vi "ET3500 - Read Program Parameters.vi"(4 "Sample/ch per Count":i32, 6 "Simulate":bool, 7 "ET3500 Status":refnum<vi>, 8 "error in (no error)":errorcluster, 9 "subVI (Auto Interactive)":bool, 10 "Option":cluster{"Init":bool, "Close":bool}={"Init"=TRUE, "Close"=TRUE}, 11 "VISA resource name":refnum<visa-resource-name>="visa://192.168.1.50/ASRL1::INSTR") -> (0 "error out":errorcluster, 1 "Segment.Type":i16=1, 2 "Parameter Cluster (Scaled)":T2={"ProgramNumber"=1, "CurProg"=33, "CurSeg"=1, "ProgStatus"=1, "ProgTimeLeft (min)"=0.0, "PVIn (degC)"=12000.0, "SPIn (NA)"=0.0, "SegTimeLeft (min)"=0.0}, 3 "VISA resource name out":refnum<visa-resource-name>="visa://192.168.1.50/ASRL1::INSTR", 5 "Segment.Duration (min)":dbl=-32768.0 format="%.2f")   [LabVIEW 2013]
uses:
  Controls/ET3500 Programmer Enum.ctl
  Controls/ET3500 Enum.ctl
  Controls/ET3500 Segment Enum.ctl
  <instrlib>/Eurotherm 35xx Series/Eurotherm 35xx Series.lvlib
panel:
  out "call chain":string[](array[string])
  out "ET3500 SegType (Simulate)":i32[](array[numeric])
  out "ET3500 Status":string="Program = 33. Segment = Rate. Status = Not running. "
  out "curSeg":T1=enum."Segment1"
  in  "stop":bool
  out "iteration":i32=11
  out "Parameter Names":T3[](array[typedef])=[0, 9, 10, 11, 17, 18, 19, 21] items=["Comms.ProgramNumber", "", "Program.RampUnits", "Program.DwellUnits", "", "", "", "", "", "Programmer.CurProg", "Programmer.CurSeg", "Programmer.ProgStatus", "", "", "", "", "", "Programmer.ProgTimeLeft", "Programmer.PVIn", "Programmer.SPIn", "", "Programmer.SegTimeLeft"]
  out "Program Parameters":i16[](array[numeric])=[1, 33, 1, 1, 0, 12000, 0, 0]
  # "visa://192.168.1.50/ASRL1::INSTR"
  # "Segment.Type\n0 - End\n1 - Rate\n3 - Dwell"
  # "ProgStatus\n1 - Not running\n2 - RUN\n4 - RUN HLD (Hold)\n8 - HLD Flashing (Holdback)"
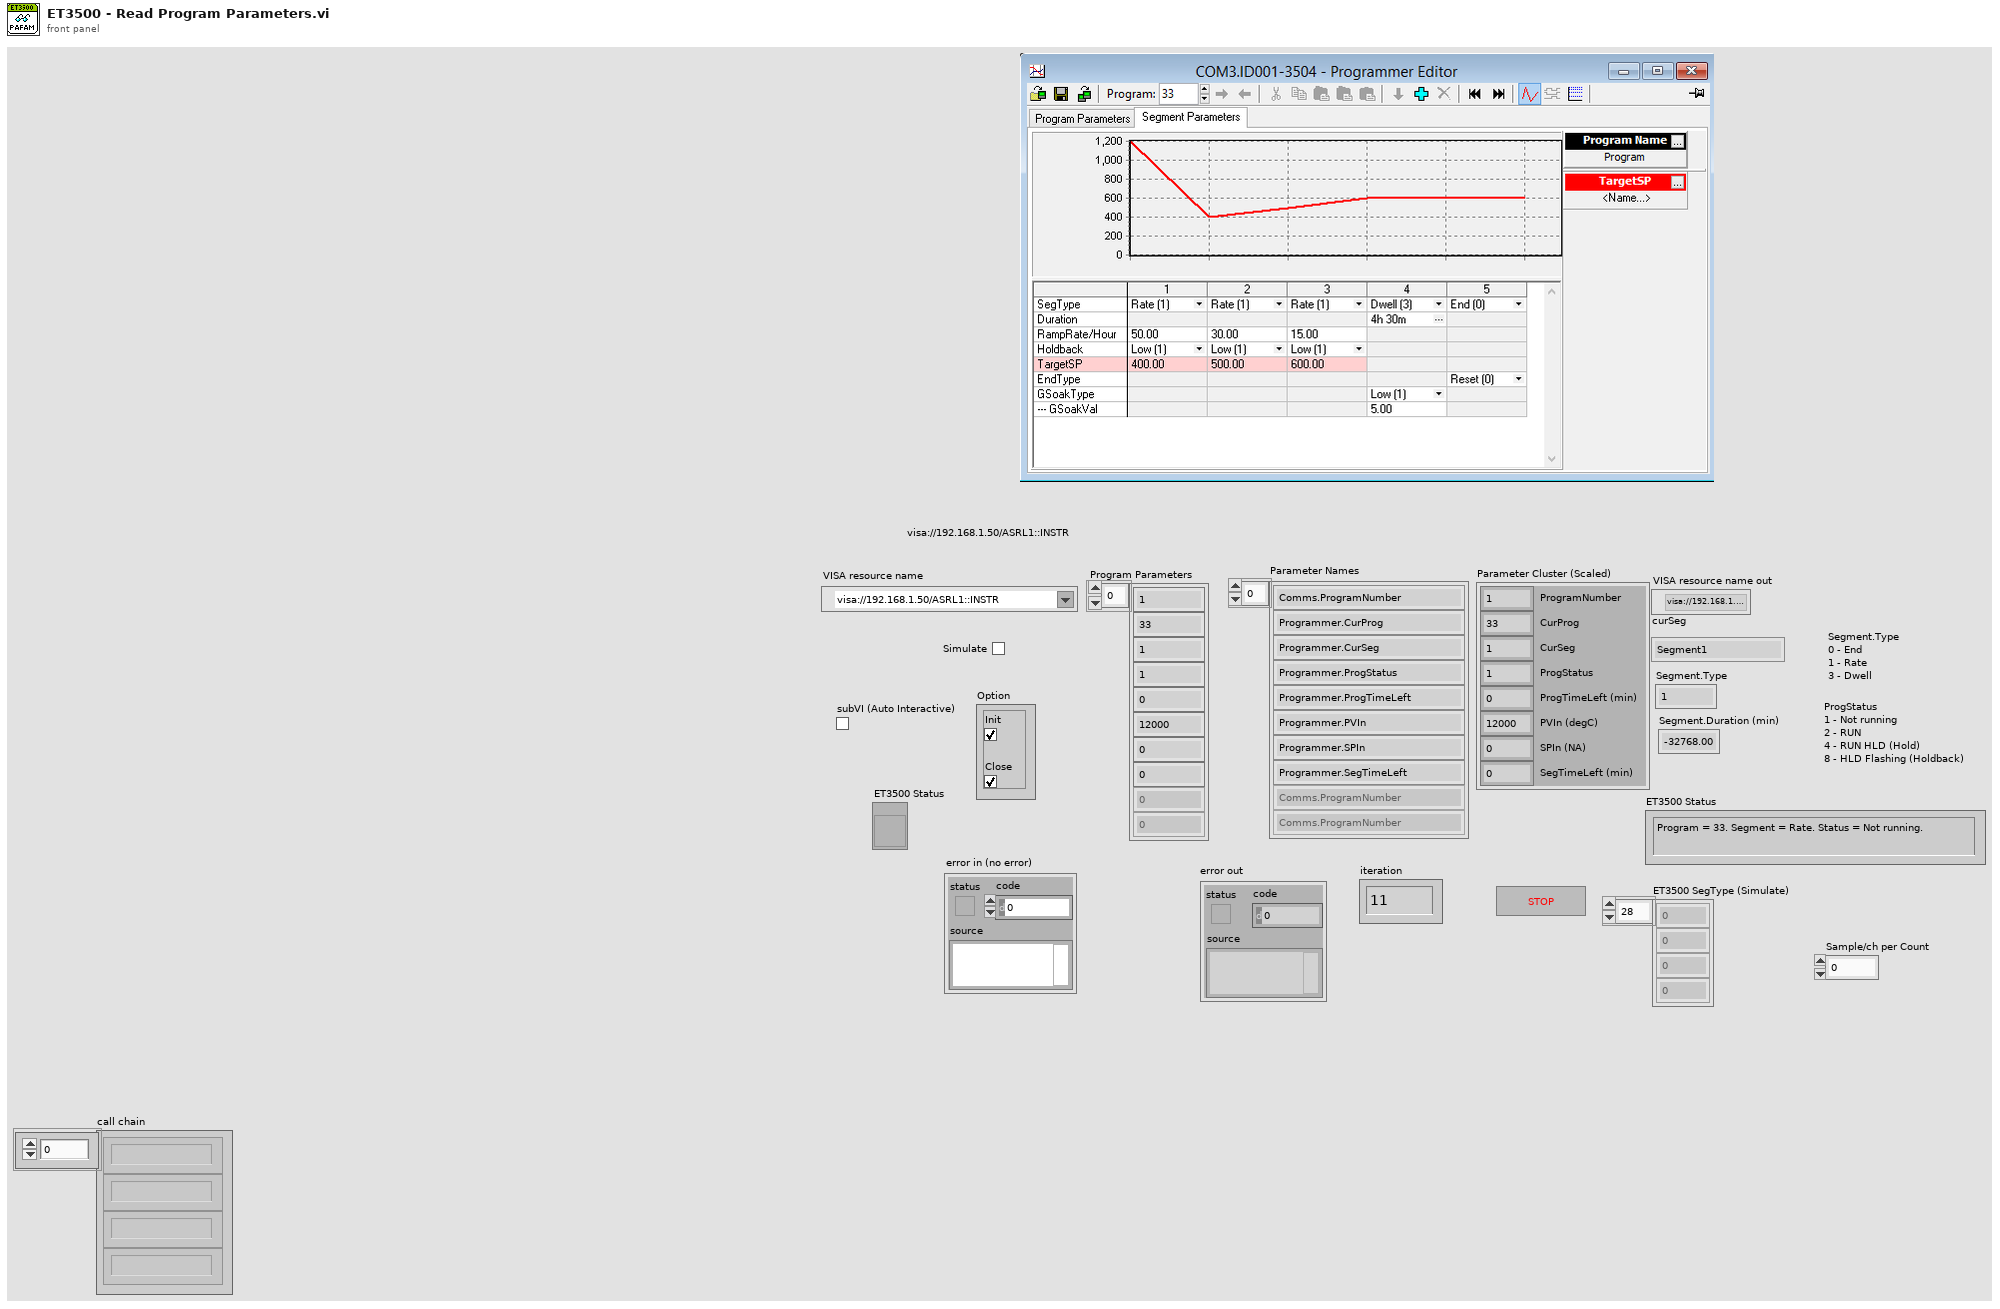
[diagram p1: front panel]
types:
  T1 = typedef "ET3500 Enum.ctl" = enum16{"Programmer1", "Segment1", "Segment2", "Segment3", "Segment4", "Segment5", "Segment6", "Segment7", "Segment8", "Segment9", "Segment10", "Segment11", "Segment12", "Segment13", "Segment14", "Segment15", "Segment16"}
  T2 = cluster{"ProgramNumber":i16, "CurProg":i16, "CurSeg":i16, "ProgStatus":i16, "ProgTimeLeft (min)":dbl, "PVIn (degC)":dbl, "SPIn (NA)":dbl, "SegTimeLeft (min)":dbl}
  T3 = typedef "ET3500 Programmer Enum.ctl" = u16
  T4 = cluster{"ProgramNumber":i16, "CurProg":i16, "CurSeg":i16, "ProgStatus":i16, "ProgTimeLeft":dbl, "PVIn":dbl, "SPIn":dbl, "SegTimeLeft":dbl}
  T5 = typedef "ET3500 Segment Enum.ctl" = u16
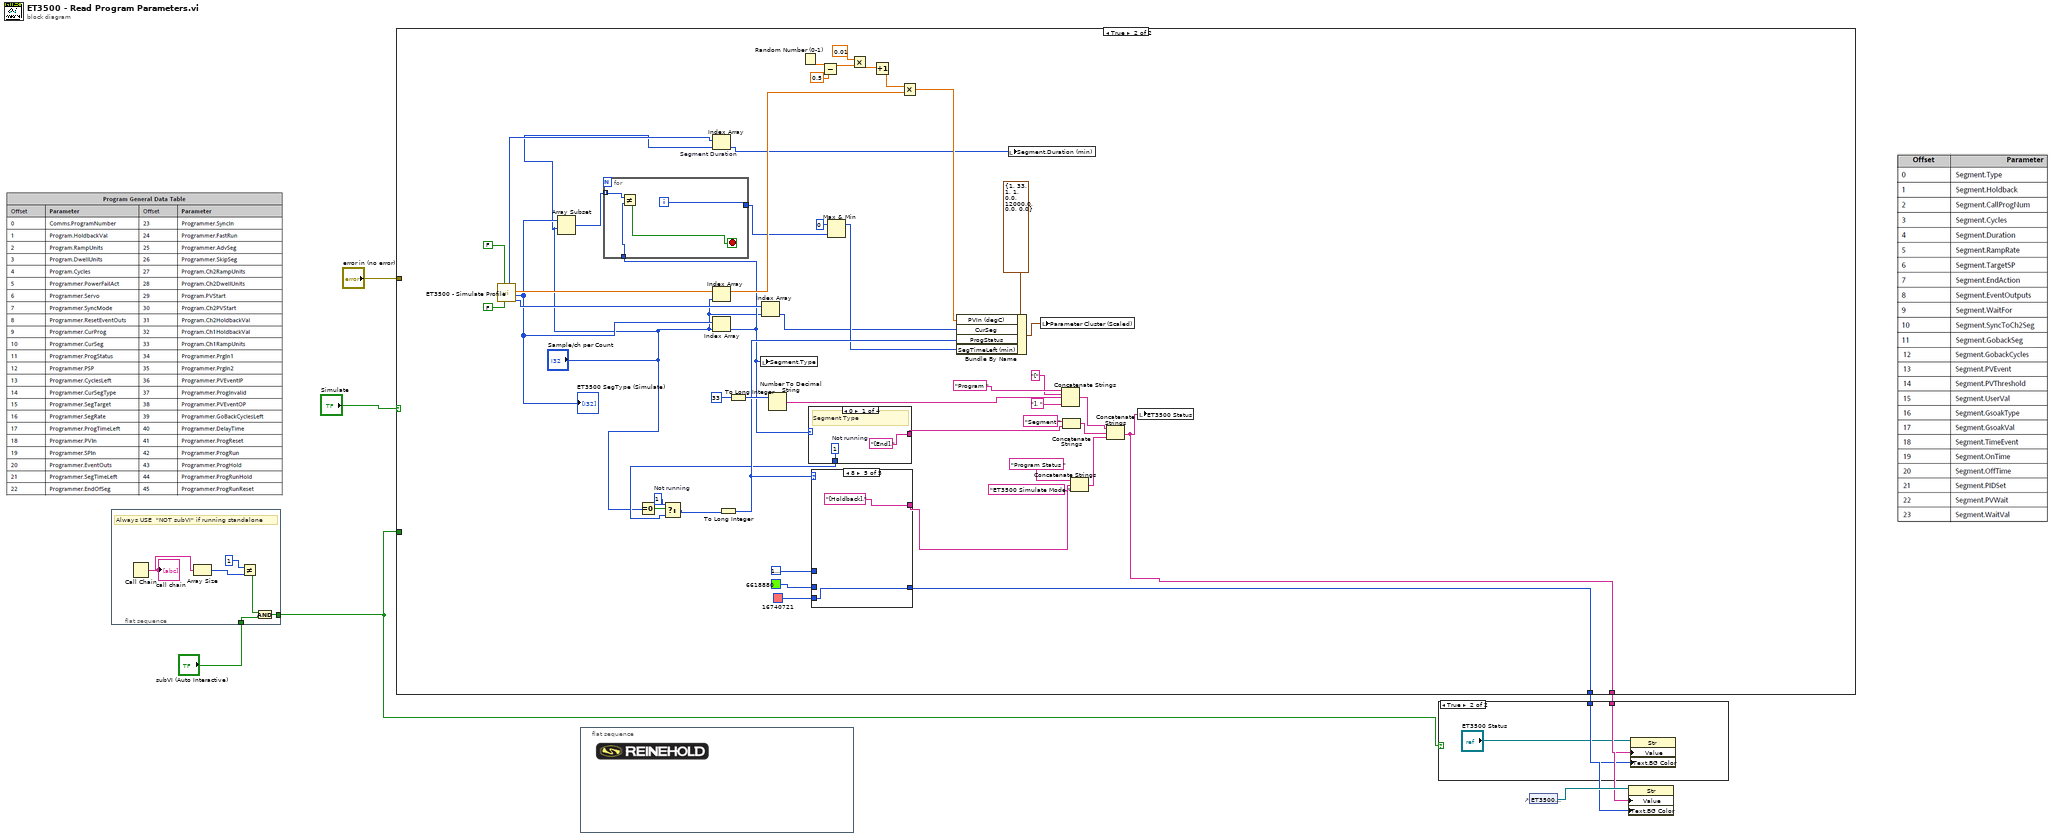
[diagram p0: block diagram]
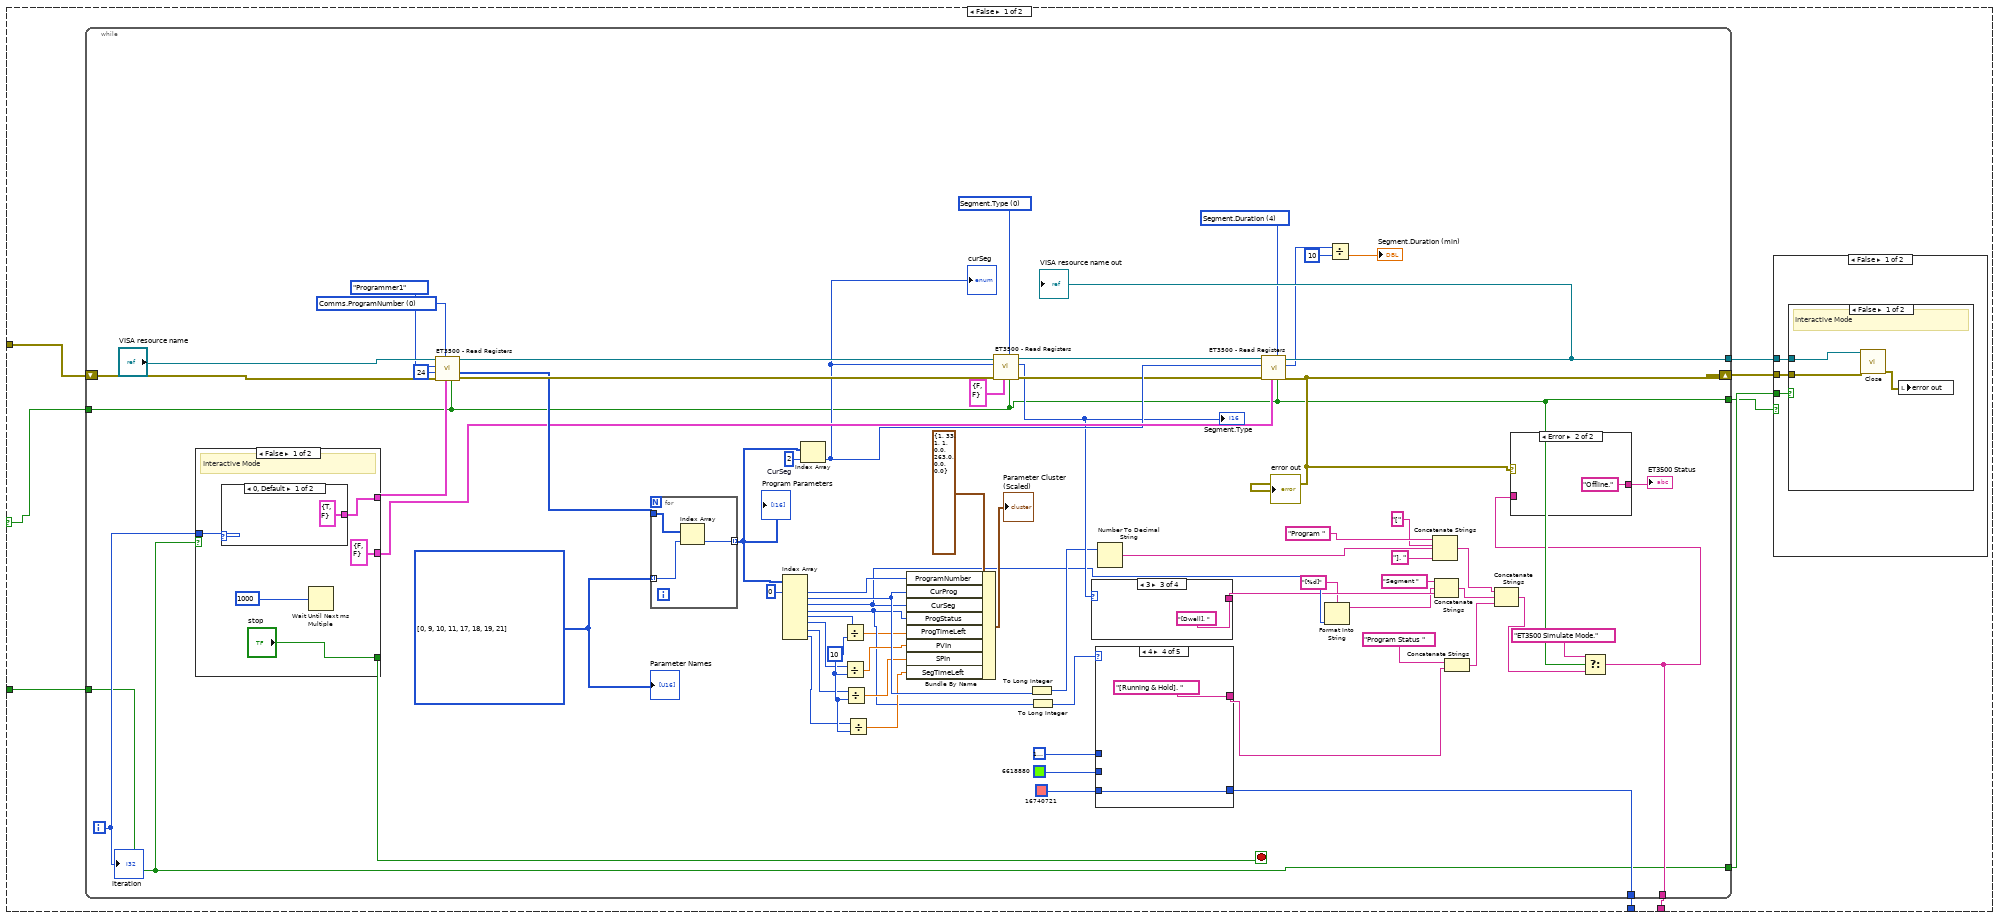
[diagram p3: hidden frame]
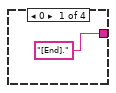
[diagram p7: hidden frame]
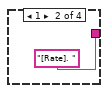
[diagram p8: hidden frame]
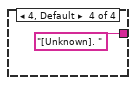
[diagram p9: hidden frame]
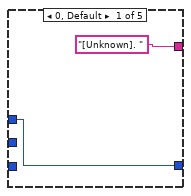
[diagram p10: hidden frame]
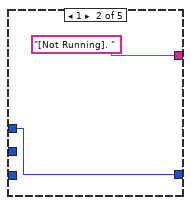
[diagram p11: hidden frame]
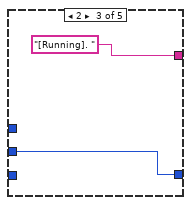
[diagram p12: hidden frame]
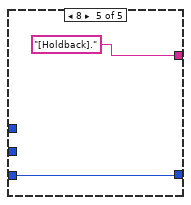
[diagram p13: hidden frame]
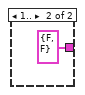
[diagram p14: hidden frame]
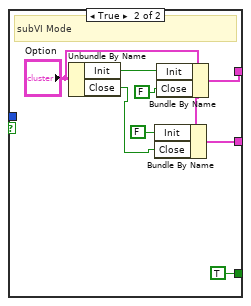
[diagram p15: hidden frame]
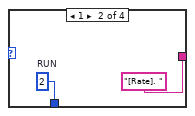
[diagram p16: hidden frame]
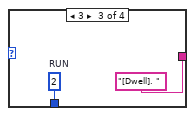
[diagram p17: hidden frame]
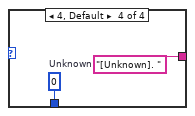
[diagram p18: hidden frame]
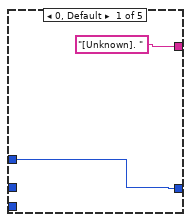
[diagram p19: hidden frame]
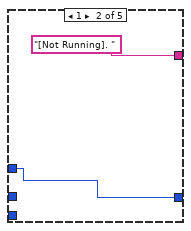
[diagram p20: hidden frame]
diagram:
  n1 = flat-sequence {
    tunnel: "subVI (Auto Interactive)" -> [w9]
    tunnel: [w8] -> w1
    frame #0 {
      # "Always USE  \"NOT subVI\" if running standalone"
      n2 = Call Chain() -> (call chain=w13:string[])
      "call chain" <- w13
      n3 = Array Size(array=w13) -> (size(s)=w12:i32)
      n4 = Not Equal?(x=1, y=w12) -> (x != y?=w11:bool)
      n5 = And(x=w11, y=w9) -> (x .and. y?=w8:bool)
    }
  }
  n6 = case shown="True" "Simulate" {
    selector: "Simulate" -> [w17 _]
    tunnel: "error in (no error)" -> [w22 _]
    tunnel: [w16 w141] -> w4
    tunnel: [w15 w140] -> w3
    tunnel: w1 -> [w14 _]
    frame False {
      n7 = while {
        shift-right: [w61] -> w20
        shift-left: w22 -> [w91]
        tunnel: [w82] -> w21
        tunnel: [w34] -> w19
        tunnel: [w40] -> w18
        tunnel: w17 -> [w40]
        tunnel: [w39] -> w16
        tunnel: [w35] -> w15
        tunnel: w14 -> [w34]
        i -> [w90]
        stop <- w84 stop-if-true
        w29 = T3[] [0, 9, 10, 11, 17, 18, 19, 21] items=["Comms.ProgramNumber", "", "Program.RampUnits", "Program.DwellUnits", "", "", "", "", "", "Programmer.CurProg", "Programmer.CurSeg", "Programmer.ProgStatus", "", "", "", "", "", "Programmer.ProgTimeLeft", "Programmer.PVIn", "Programmer.SPIn", "", "Programmer.SegTimeLeft", "Programmer.EndOfSeg", ""]
        w51 = i16 10 ("y")
        w80 = T5 4 items=["Segment.Type", "Segment.Holdback", "", "", "Segment.Duration", "Segment.RampRate", "Segment.TargetSP", "Segment.EndAction", "", "", "", "", "", "", "", "", "Segment.GsoakType", "Segment.GsoakVal"] ("ET3500 Segment Enum")
        w85 = T5 0 items=["Segment.Type", "Segment.Holdback", "", "", "Segment.Duration", "Segment.RampRate", "Segment.TargetSP", "Segment.EndAction", "", "", "", "", "", "", "", "", "Segment.GsoakType", "Segment.GsoakVal"] ("ET3500 Segment Enum")
        w86 = 2  # CurSeg
        w95 = T3 0 items=["Comms.ProgramNumber", "", "Program.RampUnits", "Program.DwellUnits", "", "", "", "", "", "Programmer.CurProg", "Programmer.CurSeg", "Programmer.ProgStatus", "", "", "", "", "", "Programmer.ProgTimeLeft", "Programmer.PVIn", "Programmer.SPIn", "", "Programmer.SegTimeLeft"] ("ET3500 Programmer Enum")
        n8 = case shown="False" w34 {
          tunnel: [w117 w126] -> w94
          tunnel: w90 -> [w116 _]
          tunnel: ["stop" TRUE ("stop")] -> w84
          tunnel: [cluster{"Init":bool, "Close":bool} {"Init"=FALSE, "Close"=FALSE} ("Option") w120] -> w81
          frame False {
            # "Interactive Mode"
            n9 = case shown="0, Default" w116 {
              tunnel: [cluster{"Init":bool, "Close":bool} {"Init"=TRUE, "Close"=FALSE} ("Option") cluster{"Init":bool, "Close":bool} {"Init"=FALSE, "Close"=FALSE} ("Option")] -> w117
              frame 0, Default {
              }
              frame 1.. {
              }
            }
            n10 = Wait Until Next ms Multiple(millisecond multiple=u32 1000) -> ()  [unwired: 1 out]
          }
          frame True {
            # "subVI Mode"
            n11 = Unbundle By Name("Option") -> ("Init"=w125:bool, "Close"=w121:bool)
            n12 = Bundle By Name(cluster="Option", "Init"=FALSE, "Close"=w121) -> (w120:cluster{"Init":bool, "Close":bool})
            n13 = Bundle By Name(cluster="Option", "Init"=w125, "Close"=FALSE) -> (w126:cluster{"Init":bool, "Close":bool})
          }
        }
        n14 = call "ET3500 - Read Registers.vi"("Simulate"=w40, "Option"=w94, "ET3500 Programmer Enum"=w95, "error in (no error)"=w91, "Num Of Reg (1)"=u16 24, "ET3500 Enum"=ET3500_Enum."Programmer1", "VISA resource name"="VISA resource name") -> ("error out"=w88:errorcluster, "Data Array"=w87:i16[], "VISA resource name out"=w89:refnum<visa-resource-name>)  [unwired: 1 in, 1 out]
        n15 = for {
          tunnel: w87 -> [w130]
          tunnel: w29 -> [w129] mode=indexing
          tunnel: [w128] -> w57 mode=indexing
          n16 = Index Array(array=w130, index=w129) -> (element=w128:i16)
        }
        "Program Parameters" <- w57
        n17 = Index Array(array=w57, index #1=0 ("index")) -> (element #1=w54:i16, element #2=w56:i16, element #3=w33:i16, element #4=w46:i16, element #5=w45:i16, element #6=w44:i16, element #7=w43:i16, element #8=w42:i16)  [unwired: 7 in]
        n18 = Index Array(array=w57, index=w86) -> (element=w79:i16)
        "curSeg" <- w79
        n19 = Divide(x=w45, y=w51) -> (x/y=w41:dbl)
        n20 = Divide(x=w44, y=w51) -> (x/y=w53:dbl)
        n21 = Divide(x=w43, y=w51) -> (x/y=w52:dbl)
        n22 = Divide(x=w42, y=w51) -> (x/y=w50:dbl)
        n23 = Bundle By Name(cluster=T4 {"ProgramNumber"=1, "CurProg"=33, "CurSeg"=1, "ProgStatus"=1, "ProgTimeLeft"=0.0, "PVIn"=263.0, "SPIn"=0.0, "SegTimeLeft"=0.0} ("Parameter Cluster"), "ProgramNumber"=w54, "CurProg"=w56, "CurSeg"=w33, "ProgStatus"=w46, "ProgTimeLeft"=w41, "PVIn"=w53, "SPIn"=w52, "SegTimeLeft"=w50) -> (→"Parameter Cluster (Scaled)":T4)
        n24 = call "ET3500 - Read Registers.vi"("Simulate"=w40, "ET3500 Segment Enum"=w85, "Option"=cluster{"Init":bool, "Close":bool} {"Init"=FALSE, "Close"=FALSE}, "error in (no error)"=w88, "ET3500 Enum"=w79, "VISA resource name"=w89) -> ("error out"=w77:errorcluster, "Data"=w75:i16, "VISA resource name out"=w83:refnum<visa-resource-name>)  [unwired: 2 in, 1 out]
        "Segment.Type" <- w75
        n25 = To Long Integer(number=w56) -> (32bit integer=w72:i32)
        n26 = To Long Integer(number=w46) -> (32bit integer=w76:i32)
        n27 = case shown="3" w75 {
          tunnel: ["[End]." "[Rate]. " "[Dwell]. " "[Unknown]. "] -> w32
          frame 0 {
          }
          frame 1 {
          }
          frame 3 {
          }
          frame 4, Default {
          }
        }
        n28 = case shown="4" w76 {
          tunnel: ["[Unknown]. " "[Not Running]. " "[Running]. " "[Running & Hold]. " "[Holdback]."] -> w68
          tunnel: u32 16777216 ("Color Box") -> [w103 w105 _ _ _]
          tunnel: [w103 w105 w107 w109 w111] -> w35
          tunnel: u32 16740721 ("Color Box") -> [_ _ _ w109 w111]
          tunnel: u32 6618880 ("Color Box") -> [_ _ w107 _ _]
          frame 0, Default {
          }
          frame 1 {
          }
          frame 2 {
          }
          frame 4 {
          }
          frame 8 {
          }
        }
        n29 = Number To Decimal String(number=w72) -> (decimal integer string=w63:string)  [unwired: 1 in]
        n30 = call "ET3500 - Read Registers.vi"("Simulate"=w40, "ET3500 Segment Enum"=w80, "Option"=w81, "error in (no error)"=w77, "ET3500 Enum"=w79, "VISA resource name"=w83) -> ("error out"=w61:errorcluster, "Data"=w48:i16, "VISA resource name out"=w82:refnum<visa-resource-name>)  [unwired: 2 in, 1 out]
        "error out" <- w61
        "VISA resource name out" <- w82
        n31 = Format Into String(format string="[%d]", w33) -> (resulting string=w31:string)  [unwired: 2 in, 1 out]
        n32 = Divide(x=w48, y=i16 10) -> (x/y=→"Segment.Duration (min)":dbl)
        n33 = Concatenate Strings("Program " ("string"), "[" ("string"), w63, "]. " ("string")) -> (w67:string)
        n34 = Concatenate Strings("Segment " ("string"), w31, w32) -> (w66:string)
        n35 = Concatenate Strings("Program Status " ("string"), w68) -> (w65:string)
        n36 = Concatenate Strings(w67, w66, w65) -> (w64:string)
        n37 = Select(t="ET3500 Simulate Mode." ("string"), s=w40, f=w64) -> (s? t:f=w39:string)
        n38 = case shown="Error" w61 {
          tunnel: w39 -> [w97 _]
          tunnel: [w97 "Offline." ("string")] -> w60
          frame No Error {
          }
          frame Error {
          }
        }
        "ET3500 Status" <- w60
        "Parameter Names" <- w29
        "iteration" <- w90
      }
      n39 = case shown="False" w18 {
        tunnel: w21 -> [w25 _]
        tunnel: w20 -> [w24 _]
        tunnel: w19 -> [w23 _]
        frame False {
          n40 = case shown="False" w23 {
            tunnel: w25 -> [w28 _]
            tunnel: w24 -> [w27 _]
            frame False {
              # "Interactive Mode"
              n41 = call <instrlib>:"Close.vi"("VISA resource name"=w28, "error in (no error)"=w27) -> ("error out"=w26:errorcluster)  [unwired: 13 in]
              n42 = local write "error out"(w26) -> ()
            }
            frame True {
              # "subVI mode"
            }
          }
        }
        frame True {
          # "Simulate"
        }
      }
    }
    frame True {
      w155 = 1  # Not running
      n43 = call "ET3500 - Simulate Profile.vi"("Popup"=FALSE, "Set (T) / Get (F)"=FALSE) -> ("Current Segment#"=w139:i32[], "ET3500 SegType"=w137:i32[], "ET3500 Profile"=w161:dbl[], "Segment Duration"=w134:i32[])  [unwired: 5 in, 1 out]
      "ET3500 SegType (Simulate)" <- w137
      n44 = Array Subset(array=w137, index="Sample/ch per Count") -> (w131:i32[])  [unwired: 1 in]
      n45 = Equal To 0?(x="Sample/ch per Count") -> (x = 0?=w156:bool)
      n46 = Index Array(array=w161, index="Sample/ch per Count") -> (element=w152:dbl)
      n47 = Index Array "Segment Duration"(array=w134, index="Sample/ch per Count") -> (element=w132:i32)
      n48 = Index Array(array=w137, index="Sample/ch per Count") -> (element=w136:i32)
      n49 = for {
        tunnel: [w180] -> w135
        tunnel: w136 -> [w181]
        tunnel: w131 -> [w182] mode=indexing
        i -> [w180]
        stop <- w179 stop-if-true
        n50 = Not Equal?(x=w182, y=w181) -> (x != y?=w179:bool)
      }
      n51 = To Long Integer(number=33) -> (32bit integer=w174:i32)
      n52 = local write "Segment.Type"(w136) -> ()
      n53 = Index Array(array=w139, index="Sample/ch per Count") -> (element=w138:i32)
      n54 = Number To Decimal String(number=w174) -> (decimal integer string=w166:string)  [unwired: 1 in]
      n55 = Random Number (0-1)() -> (number: 0 to 1=w146:dbl)
      n56 = case shown="0" w136 {
        tunnel: ["[End]." "[Rate]. " "[Dwell]. " "[Unknown]. "] -> w175
        tunnel: [w183 w185 w187 w189] -> w154
        frame 0 {
          w183 = 1  # Not running
          # "Segment Type"
        }
        frame 1 {
          w185 = 2  # RUN
        }
        frame 3 {
          w187 = 2  # RUN
        }
        frame 4, Default {
          w189 = 0  # Unknown
        }
      }
      n57 = Select(t=w155, s=w156, f=w154) -> (s? t:f=w153:i32)
      n58 = To Long Integer(number=w153) -> (32bit integer=w162:i32)
      n59 = case shown="8" w162 {
        tunnel: ["[Unknown]. " "[Not Running]. " "[Running]. " "[Running & Hold]. " "[Holdback]."] -> w170
        tunnel: [w191 w193 w195 w197 w199] -> w140
        tunnel: u32 6618880 ("Color Box") -> [_ _ w195 _ _]
        tunnel: u32 16740721 ("Color Box") -> [_ _ _ w197 w199]
        tunnel: u32 16777216 ("Color Box") -> [w191 w193 _ _ _]
        frame 0, Default {
        }
        frame 1 {
        }
        frame 2 {
        }
        frame 4 {
        }
        frame 8 {
        }
      }
      n60 = Subtract(x=w146, y=0.5) -> (x-y=w149:dbl)
      n61 = Max & Min(x=0, y=w135) -> (max(x,y)=w157:i32)  [unwired: 1 out]
      n62 = Multiply(x=0.01, y=w149) -> (x*y=w151:dbl)
      n63 = Increment(x=w151) -> (x+1=w147:dbl)
      n64 = Multiply(x=w147, y=w152) -> (x*y=w145:dbl)
      n65 = Bundle By Name(cluster=T2 {"ProgramNumber"=1, "CurProg"=33, "CurSeg"=1, "ProgStatus"=1, "ProgTimeLeft (min)"=0.0, "PVIn (degC)"=12000.0, "SPIn (NA)"=0.0, "SegTimeLeft (min)"=0.0} ("Parameter Cluster (Scaled)"), "PVIn (degC)"=w145, "CurSeg"=w138, "ProgStatus"=w162, "SegTimeLeft (min)"=w157) -> (w159:T2)
      n66 = local write "Segment.Duration (min)"(w132) -> ()
      n67 = local write "Parameter Cluster (Scaled)"(w159) -> ()
      n68 = Concatenate Strings("Program " ("string"), "[" ("string"), w166, "]. " ("string")) -> (w169:string)
      n69 = Concatenate Strings("Segment " ("string"), w175) -> (w168:string)
      n70 = Concatenate Strings("Program Status " ("string"), w170, "ET3500 Simulate Mode." ("string")) -> (w167:string)
      n71 = Concatenate Strings(w169, w168, w167) -> (w141:string)
      n72 = local write "ET3500 Status"(w141) -> ()
    }
  }
  n73 = flat-sequence {
    frame #0 {
    }
  }
  n74 = case shown="True" w1 {
    tunnel: w4 -> [_ w202]
    tunnel: w3 -> [_ w201]
    frame False {
      # "subVI"
    }
    frame True {
      n75 = property class="Str"(reference="ET3500 Status", "Value"=w202, "Text.BG Color"=w201) -> ()  [unwired: 1 in, 2 out]
    }
  }
  n76 = control-ref of="ET3500 Status"() -> (w5:refnum<vi>)
  n77 = property class="Str"(reference=w5, "Value"=w4, "Text.BG Color"=w3) -> ()  [unwired: 1 in, 2 out]
